vi "Enable Digital Port.vi"(8 "error in (no error)":errorcluster, 10 "Enable Digital Output (T: Enable)":bool=TRUE, 11 "VISA resource name":refnum<visa-resource-name>) -> (0 "error out":errorcluster, 3 "VISA resource name out":refnum<visa-resource-name>)   [LabVIEW 2021, in "Keithley 2200 Series.lvlib"]
doc: "Sets the output state of the digital port for the power supply ."
uses:
  <instrlib>/Keithley 2200 Series/Keithley 2200 Series.lvlib
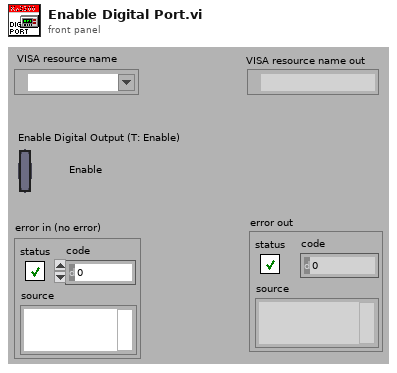
[diagram p1: front panel]
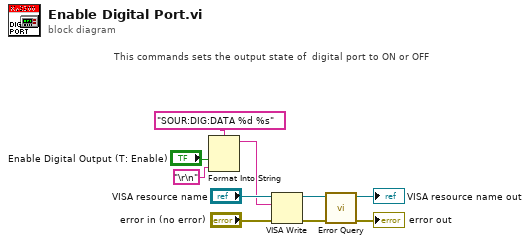
[diagram p0: block diagram]
diagram:
  # "This commands sets the output state of  digital port to ON or OFF"
  n1 = Format Into String(format string="SOUR:DIG:DATA %d %s", "Enable Digital Output (T: Enable)", "\r\n") -> (resulting string=w1:string)  [unwired: 2 in, 1 out]
  n2 = VISA Write(VISA resource name="VISA resource name", write buffer=w1, error in (no error)="error in (no error)") -> (VISA resource name out=w6:refnum<visa-resource-name>, error out=w5:errorcluster)  [unwired: 1 out]
  n3 = call <instrlib>:"Error Query.vi"("error in (no error)"=w5, "VISA resource name"=w6) -> ("error out"=→"error out":errorcluster, "VISA resource name out"=→"VISA resource name out":refnum<visa-resource-name>)  [unwired: 8 out]
